vi "~ simulation prototype subvi.vi"(11 "milliseconds to wait":u32=150) -> (3 "Motion Stopped = T":bool)   [LabVIEW 2019]
doc: "generate a random time,\nthen wait for it to expire."
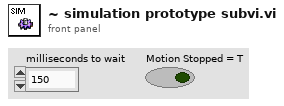
[diagram p1: front panel]
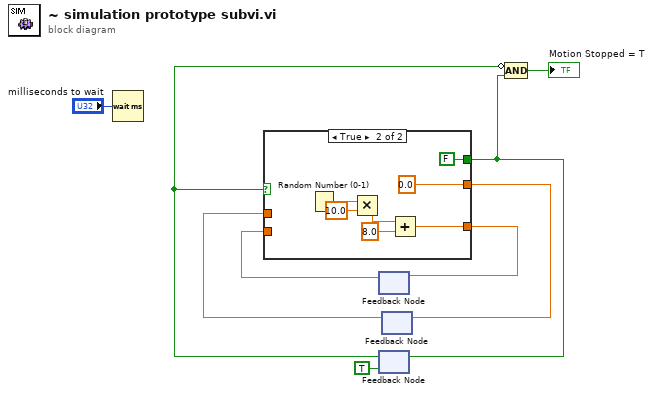
[diagram p0: block diagram]
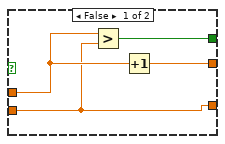
[diagram p2: hidden frame]
diagram:
  n1 = Wait (ms)(milliseconds to wait="milliseconds to wait") -> ()  [unwired: 1 out]
  n2 = feedback #1() -> (w4:dbl)  [unwired: 1 in]
  n3 = feedback #2(TRUE) -> (w7:bool)
  n4 = feedback #3() -> (w5:dbl)  [unwired: 1 in]
  n5 = case shown="True" w7 {
    tunnel: [w10 w16] -> w2
    tunnel: [w13 0.0 ("y")] -> w3
    tunnel: w4 -> [w10 _]
    tunnel: w5 -> [w12 _]
    tunnel: [w11 FALSE] -> w6
    frame False {
      n6 = Greater?(x=w12, y=w10) -> (0:w11:bool)
      n7 = Increment(x=w12) -> (x+1=w13:dbl)
    }
    frame True {
      n8 = Random Number (0-1)() -> (number: 0 to 1=w20:dbl)
      n9 = Multiply(x=w20, y=10.0) -> (x*y=w18:dbl)
      n10 = Add(x=w18, y=8.0) -> (x+y=w16:dbl)
    }
  }
  n11 = feedback-in #1(w2) -> ()
  n12 = feedback-in #2(w6) -> ()
  n13 = feedback-in #3(w3) -> ()
  n14 = Compound Arithmetic op=AND(invert w7, w6) -> (→"Motion Stopped = T":bool)
